vi "LEBITplc.MosfetSetValue.vi"(0 "i ref in":refnum<vi>, 2 "index in":i32, 3 "Special Data in":string, 5 "error in (no error)":errorcluster, 7 "element":i16, 9 "value":dbl) -> (14 "i ref out":refnum<vi>, 19 "error IO":errorcluster)   [LabVIEW 2014, in "LEBITplc.lvlib"]
uses:
  LEBITplc.lvlib
  CSlibraries-extern/DimLVEvent/LVDimInterface/LVDimInterface.lvlib
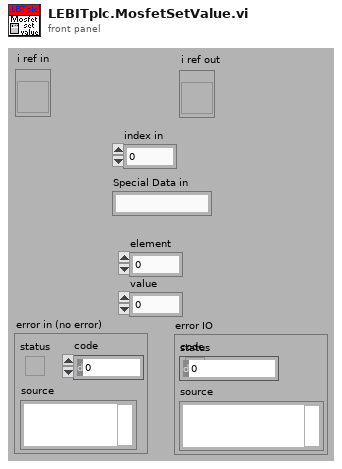
[diagram p1: front panel]
types:
  T1 = typedef "LEBITplc.lvlib/LEBITplc.i attribute.ctl" = cluster{"LLFLocation":string, "SetFileLocation":string, "nickNames":string[], "setValuePLCServiceID":i32[], "GUIServiceID":i32[], "monValuePLC":string[], "SetValueServiceID":i32[], "MonValueServiceID":i32[], "SetValue":dbl[][], "SetValueMin":dbl[], "SetValueMax":dbl[], "SetValueInfoServiceID":i32[], "GUINames":string[], "ListOfBases":string[], "Scale":dbl[], "Offset":dbl[], "setValuePLC":string[], "BaseName":string[], "ScaleServiceID":i32[], "OffsetServiceID":i32[], "AllPLCValues":string[], "CondSpecialArray":string[][], "CondSpecialIndex":i32[], "CondSpecialMonValue":dbl[], "RecentlyChanged":i32[], "SetFileLocationID":i32, "Dependent-Monitors":string[][], "LastLoadedFiles":string[], "IonGuideCalibLocation":string, "Monitor Dependent":string[], "Special":string[], "PLC?":bool[], "Start Date":string, "ListOfBasesServiceID":i32, "SETRA VISA resource":refnum<visa-resource-name>}
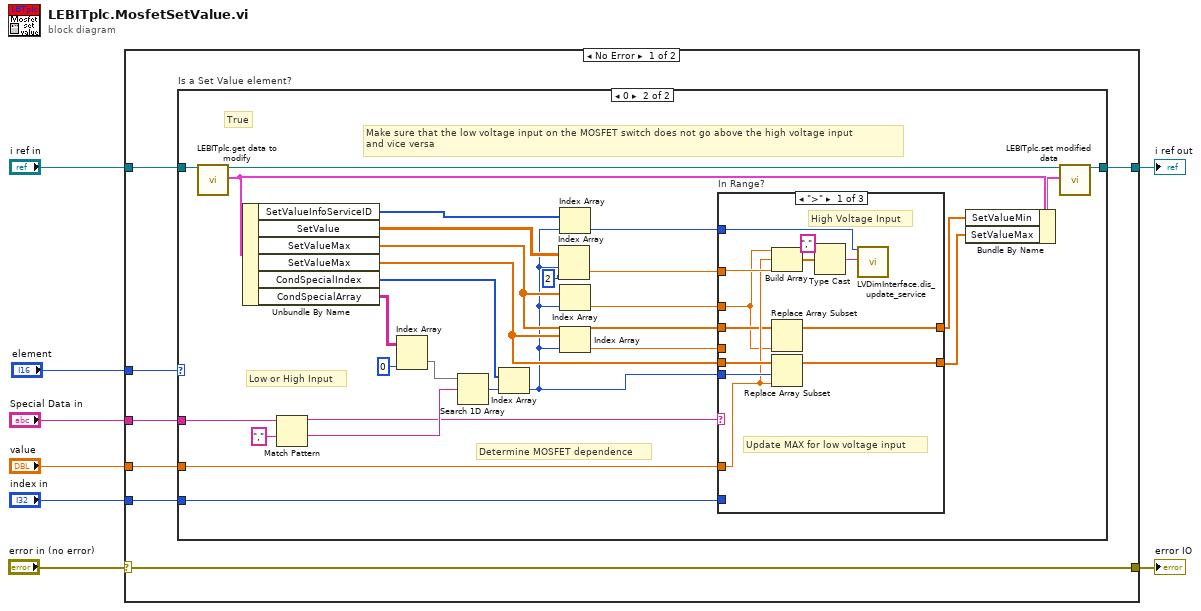
[diagram p0: block diagram]
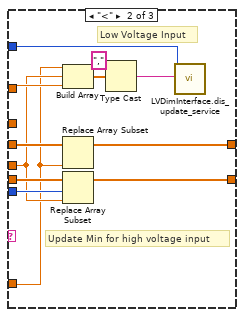
[diagram p3: hidden frame]
diagram:
  n1 = case shown="No Error" "error in (no error)" {
    selector: "error in (no error)" -> [w10 w71]
    tunnel: "value" -> [w15 _]
    tunnel: "Special Data in" -> [w14 _]
    tunnel: "index in" -> [w13 _]
    tunnel: "i ref in" -> [w12 w72]
    tunnel: [w11 w72] -> w4
    tunnel: [w10 w71] -> w2
    tunnel: "element" -> [w9 _]
    frame No Error {
      n2 = case "Is a Set Value element?" shown="0" w9 {
        tunnel: w15 -> [_ w44]
        tunnel: w14 -> [_ w40]
        tunnel: w13 -> [_ w37]
        tunnel: w12 -> [w16 w23]
        tunnel: [w16 w22] -> w11
        frame 1, Default {
          # "False"
        }
        frame 0 {
          # "True"
          # "Low or High Input"
          # "Make sure that the low voltage input on the MOSFET switch does not go above the high voltage input\nand vice versa"
          # "Determine MOSFET dependence"
          n3 = call "LEBITplc.get data to modify.vi"("i ref in"=w23) -> ("i ref out"=w24:refnum<vi>, "i attribute"=w29:T1)  [unwired: 15 in, 2 out]
          n4 = Unbundle By Name(w29) -> ("SetValueInfoServiceID"=w32:i32[], "SetValue"=w19:dbl[][], "SetValueMax"=w21:dbl[], "SetValueMax"=w35:dbl[], "CondSpecialIndex"=w41:i32[], "CondSpecialArray"=w43:string[][])
          n5 = Match Pattern(string=w40, regular expression=",") -> (before substring=w36:string, after substring=w38:string)  [unwired: 1 in, 2 out]
          n6 = Index Array(array=w43, index (col)=0 ("index (row)")) -> (element=w42:string[])  [unwired: 1 in]
          n7 = Search 1D Array(1D array=w42, element=w38) -> (index of element=w31:i32)  [unwired: 1 in]
          n8 = Index Array(array=w41, index=w31) -> (element=w18:i32)
          n9 = Index Array(array=w19, index (row)=w18, index (col)=2 ("disabled index (col)")) -> (element=w20:dbl)
          n10 = Index Array(array=w32, index=w18) -> (element=w30:i32)
          n11 = Index Array(array=w21, index=w18) -> (element=w34:dbl)
          n12 = Index Array(array=w35, index=w18) -> (element=w33:dbl)
          n13 = case "In Range?" shown="\">\"" w36 {
            tunnel: w44 -> [w48 w57 _]
            tunnel: w37 -> [_ _ _]
            tunnel: w18 -> [w55 w67 _]
            tunnel: w35 -> [w56 w68 w69]
            tunnel: w34 -> [w46 _ _]
            tunnel: w33 -> [_ w58 _]
            tunnel: w20 -> [w54 w66 _]
            tunnel: w30 -> [w50 w62 _]
            tunnel: [w49 w61 w69] -> w26
            tunnel: w21 -> [w47 w60 w70]
            tunnel: [w45 w59 w70] -> w25
            frame ">" {
              # "High Voltage Input"
              # "Update MAX for low voltage input"
              n14 = Build Array(w46, w48, w54) -> (w51:dbl[])
              n15 = Replace Array Subset(array=w47, new element=w46) -> (w45:dbl[])  [unwired: 1 in]
              n16 = Replace Array Subset(array=w56, new element=w48, index=w55) -> (w49:dbl[])
              n17 = Type Cast(type="," ("regular expression"), x=w51) -> (*(type *) &x=w53:string)
              n18 = call "LVDimInterface.dis_update_service.vi"("my_serviceID"=w50, "data"=w53) -> ()  [unwired: 15 in, 3 out]
            }
            frame "<" {
              # "Update Min for high voltage input"
              # "Low Voltage Input"
              n19 = Build Array(w57, w58, w66) -> (w63:dbl[])
              n20 = Replace Array Subset(array=w60, new element=w57) -> (w59:dbl[])  [unwired: 1 in]
              n21 = Replace Array Subset(array=w68, new element=w58, index=w67) -> (w61:dbl[])
              n22 = Type Cast(type="," ("regular expression"), x=w63) -> (*(type *) &x=w65:string)
              n23 = call "LVDimInterface.dis_update_service.vi"("my_serviceID"=w62, "data"=w65) -> ()  [unwired: 15 in, 3 out]
            }
            frame Default {
            }
          }
          n24 = Bundle By Name(cluster=w29, "SetValueMin"=w25, "SetValueMax"=w26) -> (w28:T1)
          n25 = call "LEBITplc.set modified data.vi"("i ref in"=w24, "i attribute"=w28) -> ("i ref out"=w22:refnum<vi>)  [unwired: 16 in, 1 out]
        }
      }
    }
    frame Error {
    }
  }
  "i ref out" <- w4
  "error IO" <- w2
